vi "Get SMO State.vi"(8 "error in (no error)":errorcluster, 11 "SMOFacade in":refnum<class "SMOFacade.lvclass">) -> (0 "error out":errorcluster, 2 "SMO State":T1, 3 "SMOFacade out":refnum<class "SMOFacade.lvclass">)   [LabVIEW 2013, in "SMOFacade.lvclass"]
uses:
  SMOFacade.lvclass
  SMO/Typedefs/SMOState --Enum.ctl
  SMOFacade.lvclass/SMOFacade.ctl
  SMO/SMO.lvclass
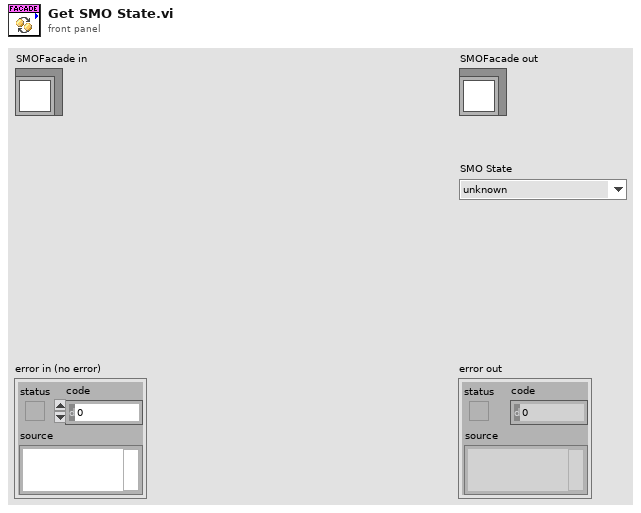
[diagram p1: front panel]
types:
  T1 = typedef "SMO.lvclass/SMOState --Enum.ctl" = enum16{"unknown", "Created", "Started", "Stopped"}
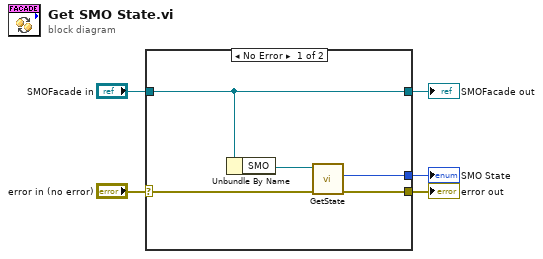
[diagram p0: block diagram]
diagram:
  n1 = case shown="No Error" "error in (no error)" {
    selector: "error in (no error)" -> [w8 w12]
    tunnel: [w7 w12] -> w4
    tunnel: [w10 w11] -> w2
    tunnel: "SMOFacade in" -> [w10 w11]
    tunnel: [w6 _] -> w1
    frame No Error {
      n2 = Unbundle By Name(w10) -> ("SMO"=w9:refnum<class "SMO.lvclass">)
      n3 = call "GetState.vi"("error in (no error)"=w8, "SMO"=w9) -> ("error out"=w7:errorcluster, "SMO State"=w6:T1)  [unwired: 7 in, 1 out]
    }
    frame Error {
    }
  }
  "error out" <- w4
  "SMOFacade out" <- w2
  "SMO State" <- w1
